vi "Error-Stop.vi"() -> ()   [LabVIEW 2020]
panel:
  in  "stop":bool
  out "error out":errorcluster
  in  "error in":errorcluster
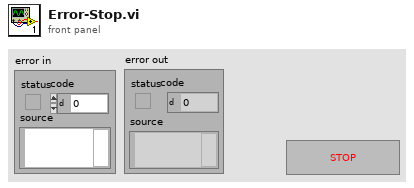
[diagram p1: front panel]
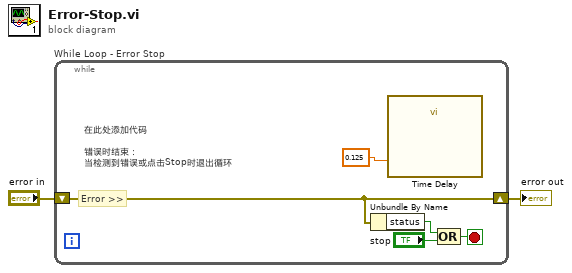
[diagram p0: block diagram]
diagram:
  n1 = while "While Loop - Error Stop" {
    shift-right: [w5] -> w1
    shift-left: "error in" -> [w5]
    stop <- w3 stop-if-true
    # "Error >>"
    # "在此处添加代码\n\n错误时结束：\n当检测到错误或点击Stop时退出循环"
    n2 = Unbundle By Name(w5) -> ("status"=w4:bool)
    n3 = call "Time Delay"("Delay Time (s)"=0.125) -> ()  [unwired: 10 in, 1 out]
    n4 = Compound Arithmetic op=OR(w4, "stop") -> (w3:bool)
  }
  "error out" <- w1
